vi "Mach_File.vi"() -> (2 "all rows":dbl[][](array[numeric]) format="%.9g", 3 "size(s)":i32[](array[numeric]))   [LabVIEW 2011]
uses:
  <vilib>/Utility/file.llb/Read Delimited Spreadsheet (DBL).vi
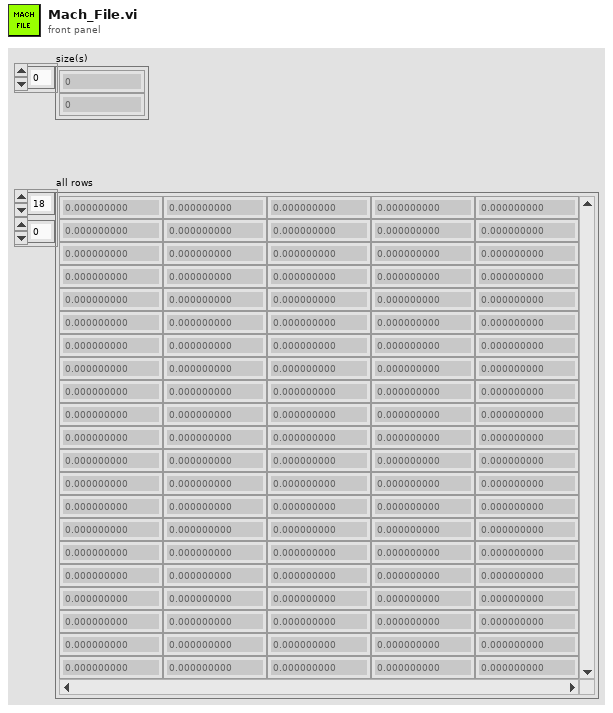
[diagram p1: front panel]
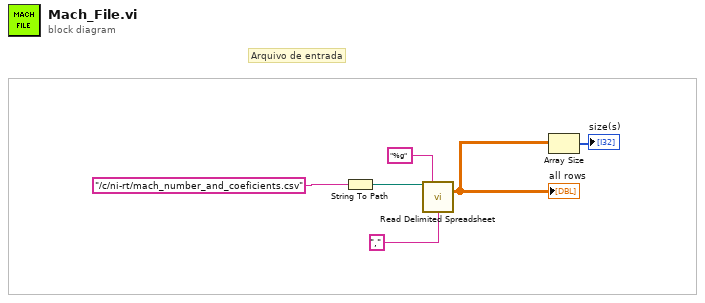
[diagram p0: block diagram]
diagram:
  # "Arquivo de entrada"
  n1 = String To Path(string="/c/ni-rt/mach_number_and_coeficients.csv" ("name or relative path")) -> (path=w1:path)
  n2 = call-poly <vilib>:"Read Delimited Spreadsheet.vi"("file path (dialog if empty)"=w1, "format (%.3f)"="%g", "delimiter (\\t)"="," ("delimiter (\\t)")) -> ("all rows"=w6:dbl[][])  [unwired: 7 in, 5 out]
  "all rows" <- w6
  n3 = Array Size(array=w6) -> (size(s)=→"size(s)":i32[])
